vi "Get References to All Libraries in Project.vi"(8 "error in":errorcluster, 11 "Project Path":path) -> (0 "error out":errorcluster, 2 "All Libraries":refnum<vi>[](array[refnum]))   [LabVIEW 2017, in "Shared Variables Library.lvlib"]
doc: "Gets references to all of the libraries, in a given project."
uses:
  Shared Variables Library.lvlib
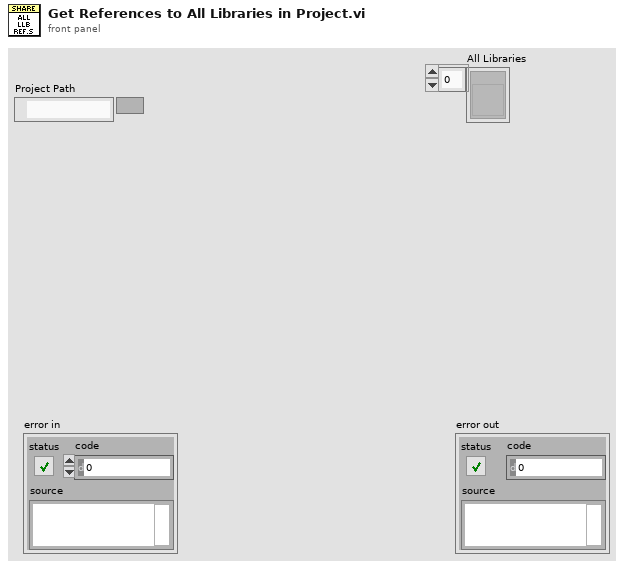
[diagram p1: front panel]
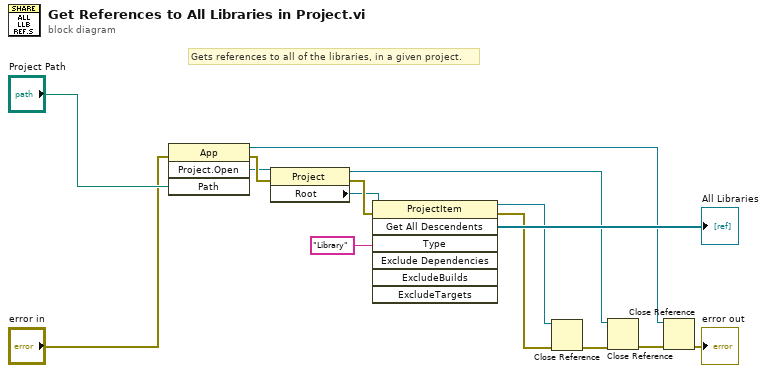
[diagram p0: block diagram]
diagram:
  # "Gets references to all of the libraries, in a given project."
  n1 = invoke class="App" method="Project.Open"(error in="error in", "Path"="Project Path") -> (reference out=w2:refnum<vi>, error out=w11:errorcluster, "Project:Open"=w10:refnum<vi>)  [unwired: 2 in, 1 out]
  n2 = property class="Project"(reference=w10, error in=w11) -> (reference out=w3:refnum<vi>, error out=w14:errorcluster, "Root"=w13:refnum<vi>)
  n3 = invoke class="ProjectItem" method="Get All Descendents"(reference=w13, error in=w14, "Type"="Library") -> (reference out=w6:refnum<vi>, error out=w7:errorcluster, "All Descendents"=→"All Libraries":refnum<vi>[])  [unwired: 4 in, 4 out]
  n4 = Close Reference(reference=w6, error in (no error)=w7) -> (error out=w5:errorcluster)
  n5 = Close Reference(reference=w3, error in (no error)=w5) -> (error out=w4:errorcluster)
  n6 = Close Reference(reference=w2, error in (no error)=w4) -> (error out=→"error out":errorcluster)
